vi "Set_subsystem_buffer.vi"(6 "channel names":string[](array[string]), 7 "Subsystem name in":string="Subsytem 1", 8 "error in (no error)":errorcluster, 10 "Buffer size":dbl=50.0, 11 "Refnum in":refnum<k34>) -> (0 "error out":errorcluster, 3 "Refnum out":refnum<k34>)   [LabVIEW 2017, in "labview-standard-library.lvlib"]
uses:
  labview-standard-library.lvlib
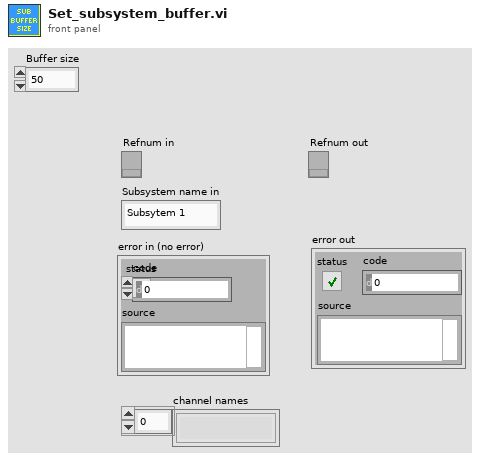
[diagram p1: front panel]
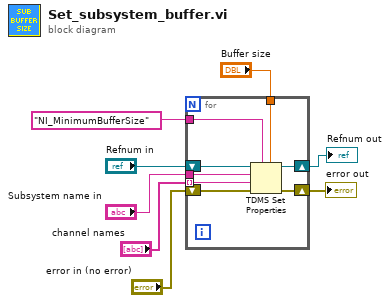
[diagram p0: block diagram]
diagram:
  n1 = for {
    tunnel: "Subsystem name in" -> [w15]
    tunnel: "Buffer size" -> [w13]
    tunnel: "NI_MinimumBufferSize" -> [w12]
    tunnel: "channel names" -> [w9] mode=indexing
    shift-right: [w14] -> w6
    shift-left: "Refnum in" -> [w16]
    shift-right: [w11] -> w4
    shift-left: "error in (no error)" -> [w10]
    n2 = TDMS Set Properties(5:w13, 7:w12, 8:w10, 9:w9, 10:w15, 11:w16) -> (0:w11:errorcluster, 3:w14:refnum<k34>)  [unwired: 2 out]
  }
  "Refnum out" <- w6
  "error out" <- w4
